vi "Plotar gráfico edição.vi"(7 "Enum":enum16{"set", "get"}(ring)=enum."get", 8 "error in (no error)":errorcluster, 11 "Entrada Cluster de onda":waveform(dbl)(graph)) -> (0 "error out":errorcluster, 3 "Plot":waveform(dbl)(graph))   [LabVIEW 2020]
doc: "Gets the plot data or Sets the FGV value with new data. used to pass data to the HTTP Method"
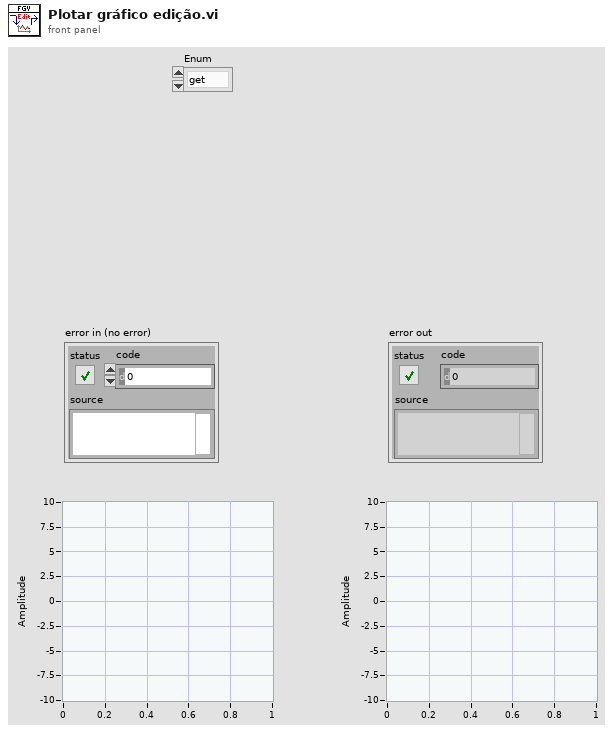
[diagram p1: front panel]
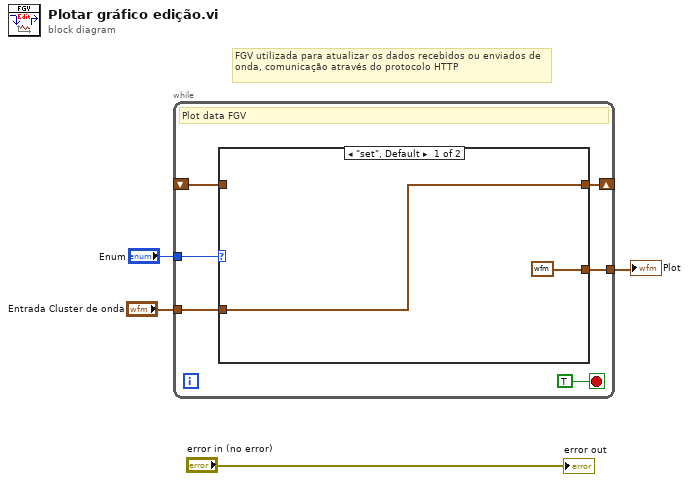
[diagram p0: block diagram]
diagram:
  # "FGV utilizada para atualizar os dados recebidos ou enviados de onda, comunicação através do protocolo HTTP"
  n1 = while {
    shift-right: [w10] -> _
    shift-left: _ -> [w9]
    tunnel: "Enum" -> [w8]
    tunnel: [w7] -> w1
    tunnel: "Entrada Cluster de onda" -> [w6]
    stop <- TRUE stop-if-true
    # "Plot data FGV"
    n2 = case shown="\"set\", Default" w8 {
      tunnel: [w12 w13] -> w10
      tunnel: w9 -> [_ w13]
      tunnel: [waveform(dbl) {"t0"=timestamp(0 s since 1904-01-01), "dt"=1.0, "Y"=[]} ("Plot 2") w13] -> w7
      tunnel: w6 -> [w12 _]
      frame "set", Default {
      }
      frame "get" {
      }
    }
  }
  "Plot" <- w1
  "error out" <- "error in (no error)"
